vi "WriteExp.vi"(8 "error in (no error)":errorcluster, 9 "Control Task In":refnum<k21>, 10 "Waveform Task In":refnum<k21>, 11 "Experimental Control Cluster In":T2) -> (0 "error out":errorcluster, 1 "waveform task out":refnum<k21>, 2 "counter task out":refnum<k21>, 3 "Experimental Control Cluster Out":T2)   [LabVIEW 2013]
uses:
  6704/6704_static_voltages_control.ctl
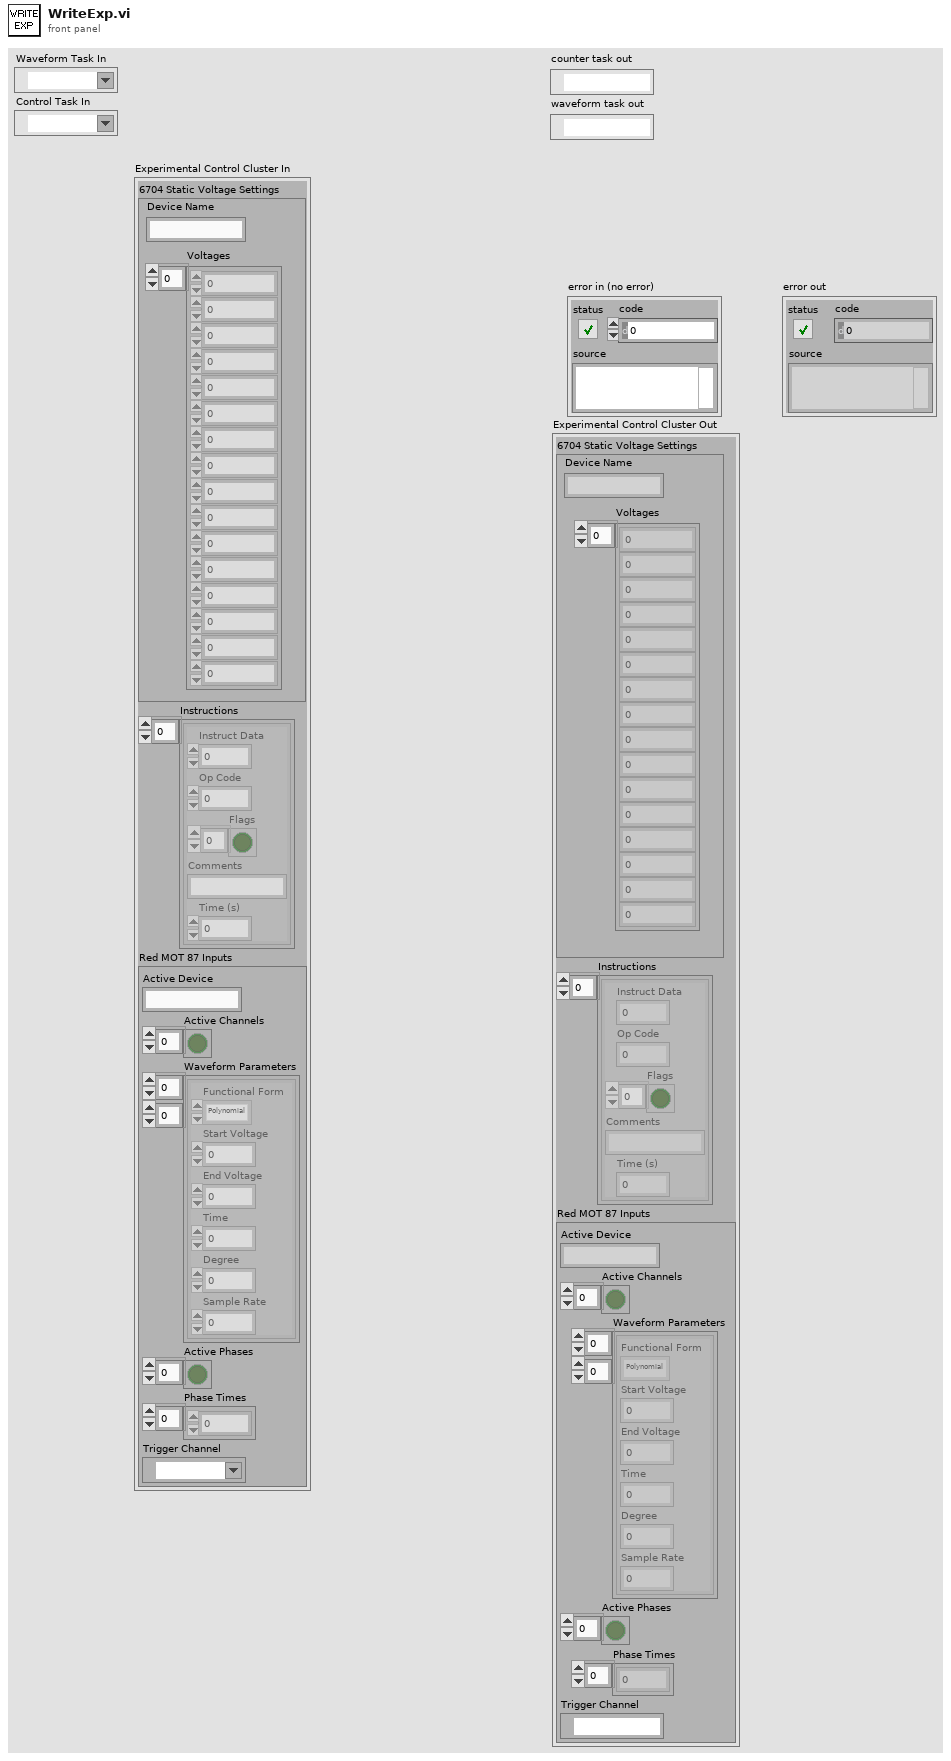
[diagram p1: front panel]
types:
  T1 = typedef "6704_static_voltages_control.ctl" = cluster{"Device Name":string, "Voltages":dbl[]}
  T2 = cluster{"6704 Static Voltage Settings":T1, "Instructions":cluster{"Instruct Data":i32, "Op Code":i32, "Flags":bool[], "Comments":string, "Time (s)":dbl}[], "Red MOT 87 Inputs":cluster{"Active Device":string, "Active Channels":bool[], "Waveform Parameters":cluster{"Functional Form":enum16{"Polynomial", "Exponential"}, "Start Voltage":dbl, "End Voltage":dbl, "Time":dbl, "Degree":i8, "Sample Rate":dbl}[][], "Active Phases":bool[], "Phase Times":dbl[], "Trigger Channel":tag}}
  T3 = enum16{"Pulse Program", "Frequency Registers", "TX Phase Registers", "RX Phase Registers"}
  T4 = cluster{"Instruct Data":i32, "Op Code":i32, "Flags":bool[], "Comments":string, "Time (s)":dbl}[]
  T5 = cluster{"Active Device":string, "Active Channels":bool[], "Waveform Parameters":cluster{"Functional Form":enum16{"Polynomial", "Exponential"}, "Start Voltage":dbl, "End Voltage":dbl, "Time":dbl, "Degree":i8, "Sample Rate":dbl}[][], "Active Phases":bool[], "Phase Times":dbl[], "Trigger Channel":tag}
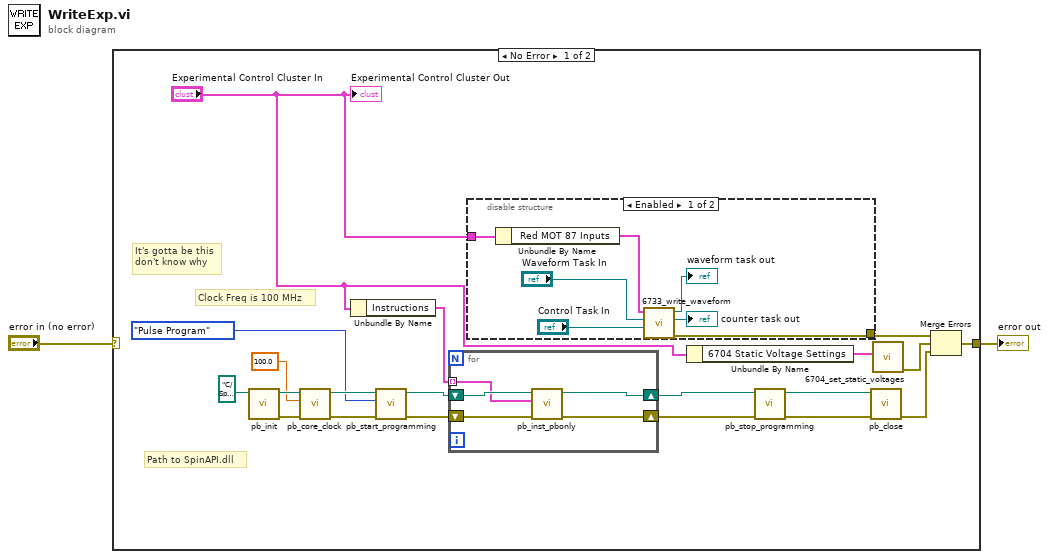
[diagram p0: block diagram]
diagram:
  n1 = case shown="No Error" "error in (no error)" {
    selector: "error in (no error)" -> [_ w35]
    tunnel: [w7 w35] -> w1
    frame No Error {
      # "It's gotta be this\ndon't know why"
      # "Clock Freq is 100 MHz"
      # "Path to SpinAPI.dll"
      n2 = call "pb_init.vi"("path in"=path "C:/SpinCore/SpinAPI/lib32/spinapi.dll") -> ("error out"=w20:errorcluster, "path out"=w19:path)  [unwired: 3 in, 6 out]
      n3 = call "pb_core_clock.vi"("error in (no error)"=w20, "clock_freq (MHz)"=100.0, "path in"=w19) -> ("error out"=w17:errorcluster, "path out"=w16:path)  [unwired: 7 in]
      n4 = Unbundle By Name("Experimental Control Cluster In") -> ("Instructions"=w14:T4)
      n5 = call "pb_start_programming.vi"("error in (no error)"=w17, "Device"=T3."Pulse Program", "path in"=w16) -> ("error out"=w13:errorcluster, "path out"=w12:path)  [unwired: 1 in, 6 out]
      n6 = for {
        tunnel: w14 -> [w31] mode=indexing
        shift-right: [w33] -> w10
        shift-left: w12 -> [w34]
        shift-right: [w30] -> w11
        shift-left: w13 -> [w32]
        n7 = call "pb_inst_pbonly.vi"("error in (no error)"=w32, "PB Instruction"=w31, "path in"=w34) -> ("error out"=w30:errorcluster, "path out"=w33:path)  [unwired: 2 in, 5 out]
      }
      n8 = disable-structure shown="Enabled" {
        disable-tunnel: "Experimental Control Cluster In" -> [w29 _]
        disable-tunnel: [w27 _] -> w3
        frame Enabled {
          n9 = Unbundle By Name(w29) -> ("Red MOT 87 Inputs"=w28:T5)
          n10 = call "6733_write_waveform.vi"("Control Task In"="Control Task In", "Waveform Task In"="Waveform Task In", "Inputs"=w28) -> ("error out"=w27:errorcluster, "counter task out"=→"counter task out":refnum<k21>, "waveform task out"=→"waveform task out":refnum<k21>)  [unwired: 6 in]
        }
        frame Disabled {
        }
      }
      n11 = Unbundle By Name("Experimental Control Cluster In") -> ("6704 Static Voltage Settings"=w22:T1)
      n12 = call "pb_stop_programming.vi"("error in (no error)"=w11, "path in"=w10) -> ("error out"=w5:errorcluster, "path out"=w6:path)  [unwired: 1 in, 7 out]
      n13 = call "pb_close.vi"("error in (no error)"=w5, "path in"=w6) -> ("error out"=w9:errorcluster)  [unwired: 9 out]
      n14 = call "6704_set_static_voltages.vi"("6704 Static Voltage Settings"=w22) -> ("error out"=w8:errorcluster)  [unwired: 7 in, 1 out]
      n15 = Merge Errors(w3, w8, w9) -> (w7:errorcluster)
      "Experimental Control Cluster Out" <- "Experimental Control Cluster In"
    }
    frame Error {
    }
  }
  "error out" <- w1
